vi "Events to table.vi"(8 "error in":errorcluster, 11 "All Events":set{T1}(c389)) -> (0 "error out":errorcluster, 3 "Table Control":string[][](table))   [LabVIEW 2019]
uses:
  Logger_class/EventData.ctl
  Logger_class/EventCode.ctl
  Logger_class/Priority.ctl
  Logger_class/Logger.lvclass
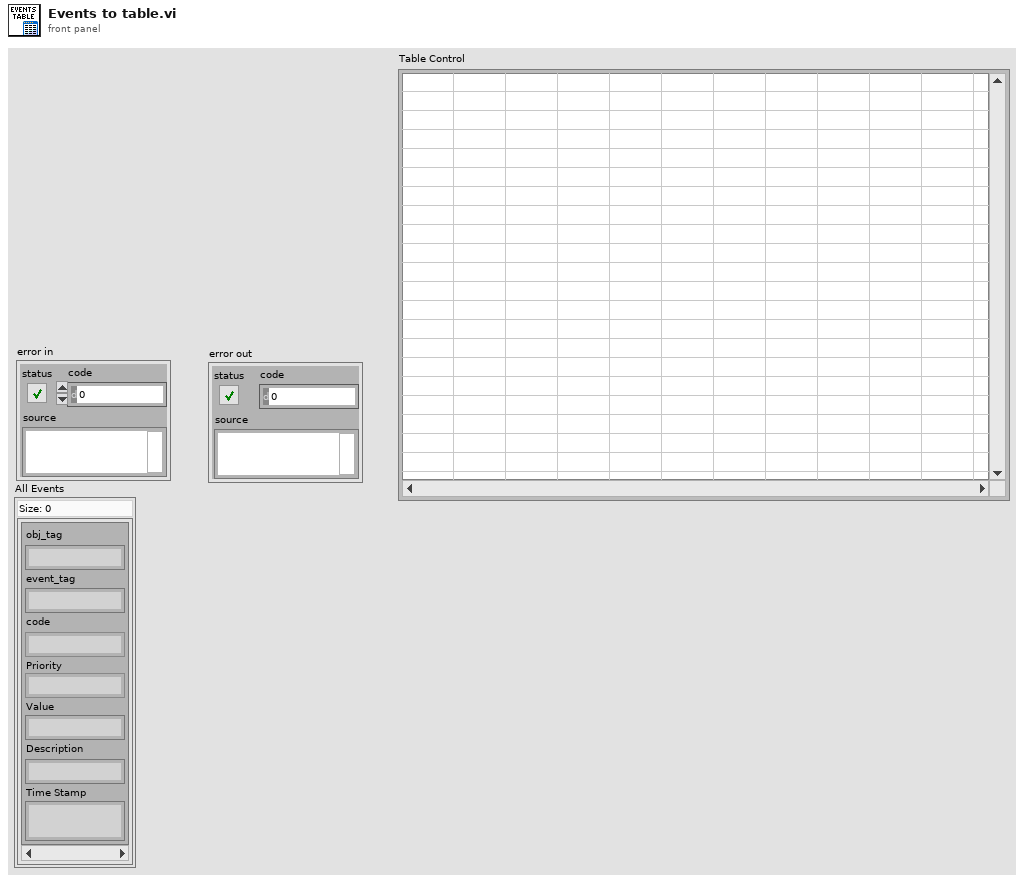
[diagram p1: front panel]
types:
  T1 = typedef "Logger.lvclass/EventData.ctl" = cluster{"obj_tag":string, "event_tag":string, "code":T2, "Priority":T3, "Value":dbl, "Description":string, "Time Stamp":timestamp}
  T2 = typedef "Logger.lvclass/EventCode.ctl" = enum16{"DI_EU_LO", "DI_EU_HI", "DIO_LO", "DIO_HI", "DI_RAW_LO", "DI_RAW_HI", "DO_LO", "DO_HI", "DA_OK", "DA_ALARM", "AA_HI", "AA_HIHI", "AA_LO", "AA_LOLO", "AA_OK", "CMD", "OUT_OF_RANGE_OK", "OUT_OF_RANGE_LO", "OUT_OF_RANGE_HI", "CONFIG", "DI_LO", "DI_HI"}
  T3 = typedef "Logger.lvclass/Priority.ctl" = enum16{"Alert", "Critical", "Error", "Warning", "Notice", "Informational", "Debug"}
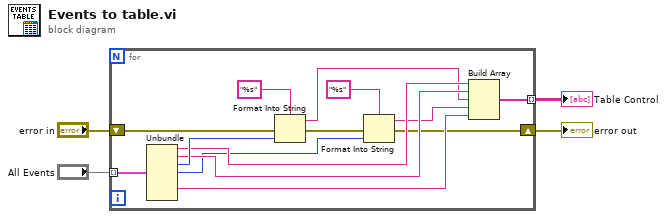
[diagram p0: block diagram]
diagram:
  n1 = for {
    tunnel: "All Events" -> [w18] mode=indexing
    tunnel: [w12] -> w4 mode=indexing
    shift-right: [w6] -> w2
    shift-left: "error in" -> [w5]
    n2 = Unbundle(w18) -> ("obj_tag"=w15:string, "event_tag"=w14:string, "code"=w17:T2, "Priority"=w10:T3, "Description"=w8:string)  [unwired: 2 out]
    n3 = Format Into String(format string="%s", error in=w5, w17) -> (resulting string=w13:string, error out=w7:errorcluster)  [unwired: 1 in]
    n4 = Format Into String(format string="%s", error in=w7, w10) -> (resulting string=w9:string, error out=w6:errorcluster)  [unwired: 1 in]
    n5 = Build Array(w15, w14, w13, w9, w8) -> (w12:string[])
  }
  "Table Control" <- w4
  "error out" <- w2
